vi "Configure Envelope.vi"(0 "VISA resource name":refnum<visa-resource-name>, 5 "Limit Line (1)":i32=1 min=1 max=6, 7 "Envelope Points (41)":i32=41 min=2 max=100, 9 "Offset Level (3.00dB)":dbl=3.0 min=-300.0 max=300.0, 11 "error in (no error)":errorcluster, 12 "Shape (1:Slope)":i32(ring)=1 items=["Square", "Slope"]) -> (4 "VISA resource name out":refnum<visa-resource-name>, 15 "error out":errorcluster)   [LabVIEW 2020, in "Anritsu Signal Analyzer Series.lvlib"]
doc: "Configures the envelope settings of the spectrum analyzer."
uses:
  Anritsu Signal Analyzer Series.lvlib
panel:
  # "dB"
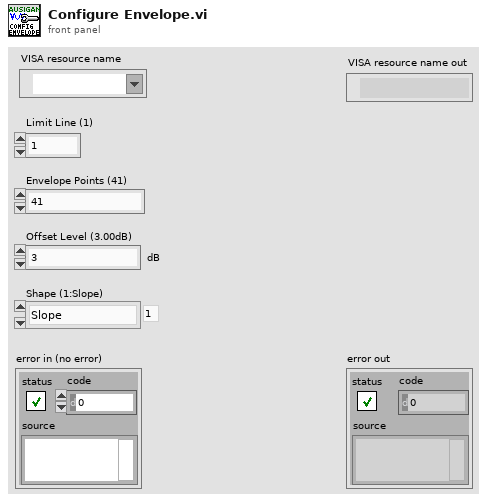
[diagram p1: front panel]
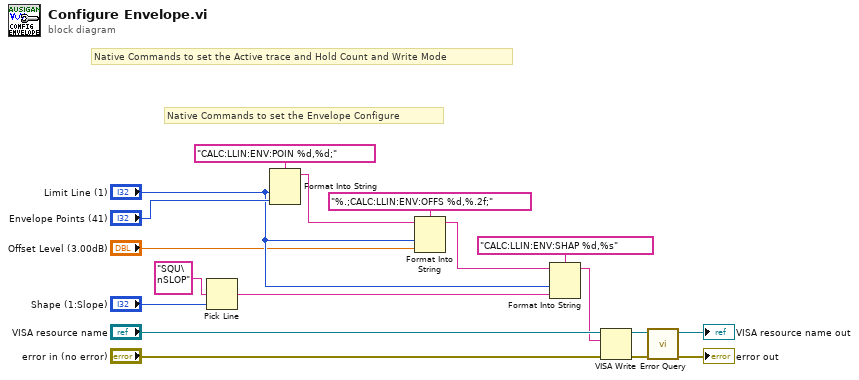
[diagram p0: block diagram]
diagram:
  # "Native Commands to set the Envelope Configure"
  # "Native Commands to set the Active trace and Hold Count and Write Mode"
  n1 = Pick Line(multi-line string="SQU\nSLOP" ("複数行文字列"), line index="Shape (1:Slope)") -> (output string=w10:string)  [unwired: 1 in]
  n2 = Format Into String(format string="CALC:LLIN:ENV:POIN %d,%d;", "Limit Line (1)", "Envelope Points (41)") -> (resulting string=w3:string)  [unwired: 2 in, 1 out]
  n3 = Format Into String(format string="%.;CALC:LLIN:ENV:OFFS %d,%.2f;", initial string=w3, "Limit Line (1)", "Offset Level (3.00dB)") -> (resulting string=w8:string)  [unwired: 1 in, 1 out]
  n4 = Format Into String(format string="CALC:LLIN:ENV:SHAP %d,%s", initial string=w8, "Limit Line (1)", w10) -> (resulting string=w7:string)  [unwired: 1 in, 1 out]
  n5 = VISA Write(VISA resource name="VISA resource name", write buffer=w7, error in (no error)="error in (no error)") -> (VISA resource name out=w14:refnum<visa-resource-name>, error out=w13:errorcluster)  [unwired: 1 out]
  n6 = call "Error Query.vi"("error in (no error)"=w13, "VISA resource name"=w14) -> ("error out"=→"error out":errorcluster, "VISA resource name out"=→"VISA resource name out":refnum<visa-resource-name>)  [unwired: 6 in, 2 out]
